vi "get valid output path.vi"(8 "error in (no error)":errorcluster, 11 "TDMS datalogger configuration in":refnum<class "TDMS datalogger configuration.lvclass">) -> (0 "error out":errorcluster, 2 "Path":path, 3 "TDMS datalogger configuration out":refnum<class "TDMS datalogger configuration.lvclass">)   [LabVIEW 2013, in "TDMS datalogger configuration.lvclass"]
uses:
  TDMS datalogger configuration.lvclass
  TDMS datalogger configuration.lvclass/TDMS datalogger configuration.ctl
  <vilib>/NI/Configuration Framework/serializable configuration/NISE_CEF_serializable configuration.lvclass/NISE_CEF_serializable configuration.ctl
  <vilib>/NI/Configuration Framework/serializable configuration/NISE_CEF_serializable configuration.lvclass
  Read Path.vi
  <vilib>/NI/Configuration Framework/serializable configuration/Read UID.vi
panel:
  out "group":string
  out "owner":string
  out "Boolean array":bool[](array[boolean])
  out "permissions":i16
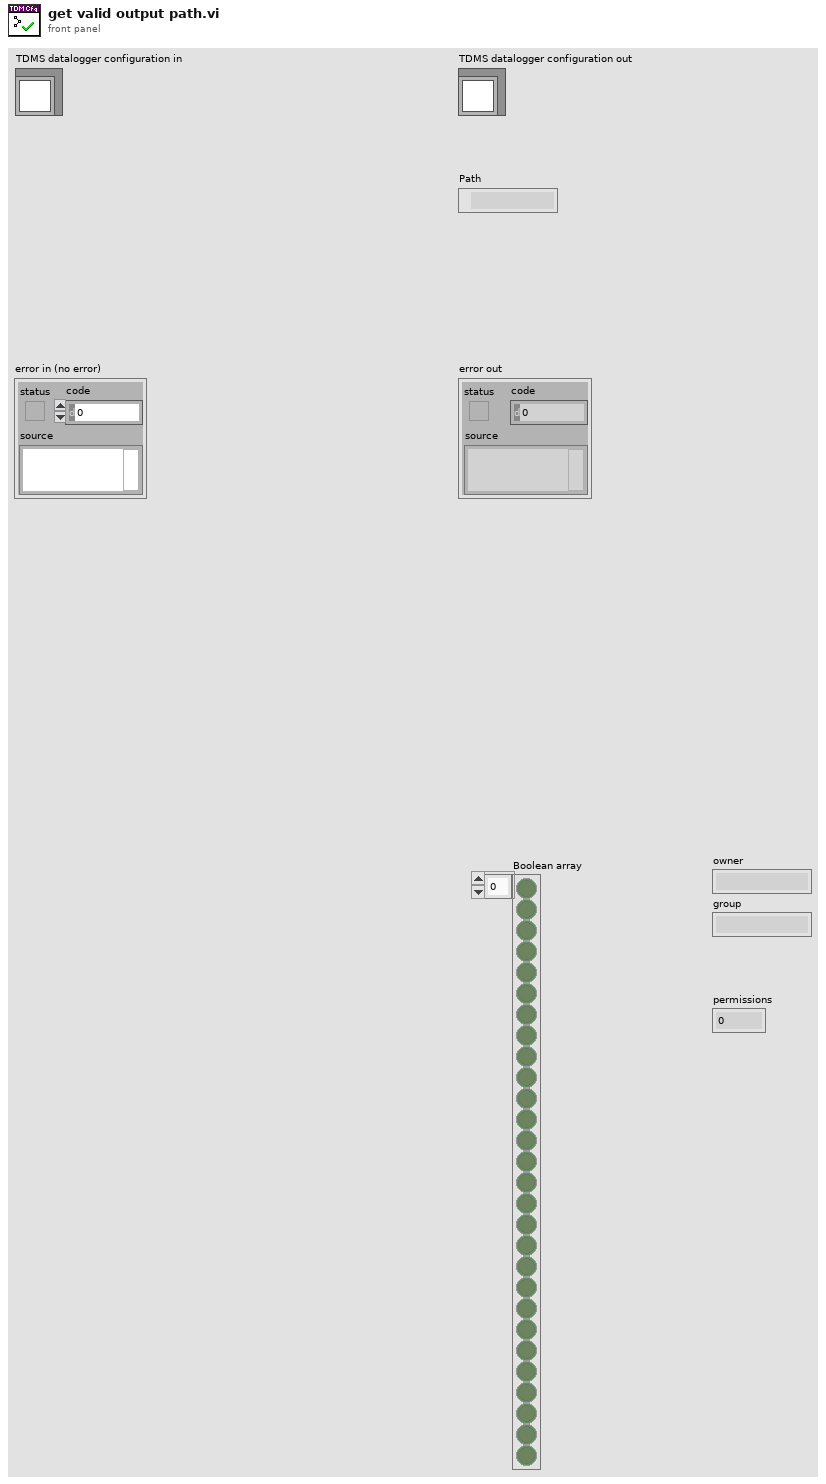
[diagram p1: front panel]
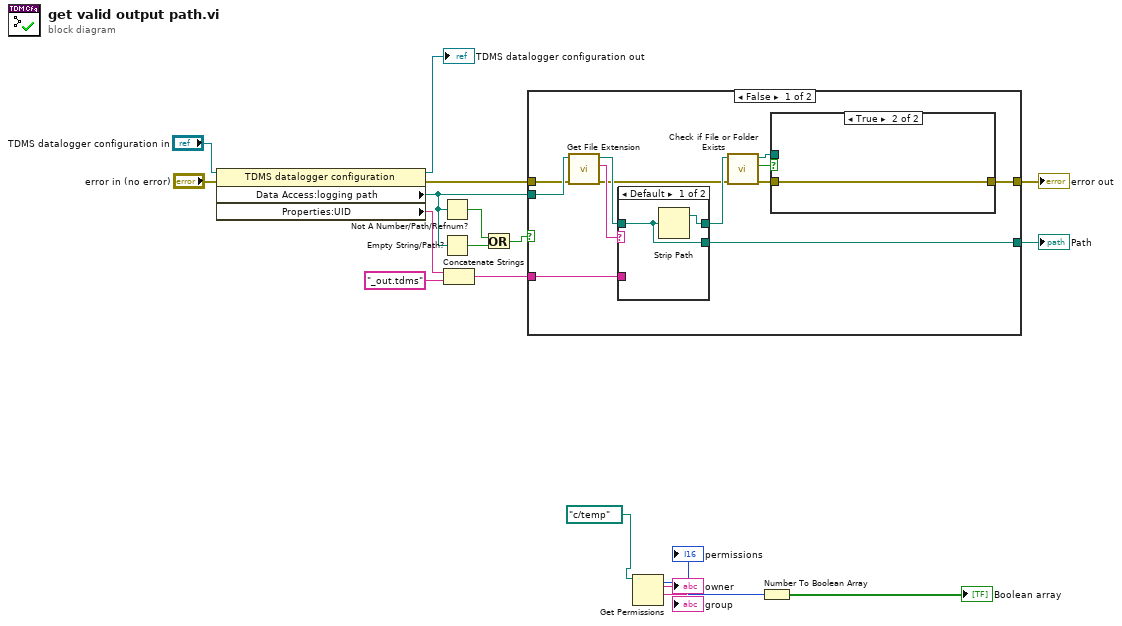
[diagram p0: block diagram]
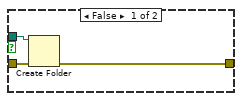
[diagram p2: hidden frame]
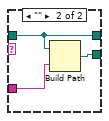
[diagram p3: hidden frame]
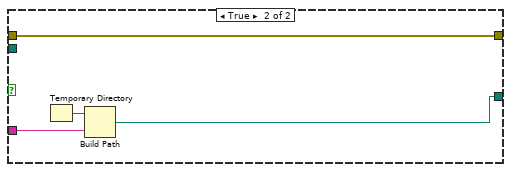
[diagram p4: hidden frame]
diagram:
  n1 = property class="TDMS datalogger configuration"(reference="TDMS datalogger configuration in", error in="error in (no error)") -> (reference out=→"TDMS datalogger configuration out":refnum<class "TDMS datalogger configuration.lvclass">, error out=w15:errorcluster, "Data Access:logging path"=w6:path, "Properties:UID"=w13:string)
  n2 = Not A Number/Path/Refnum?(number/path/refnum=w6) -> (NaN/Path/Refnum?=w17:bool)
  n3 = Empty String/Path?(string/path=w6) -> (empty?=w18:bool)
  n4 = Concatenate Strings(w13, "_out.tdms" ("string")) -> (w12:string)
  n5 = Or(x=w17, y=w18) -> (x .or. y?=w16:bool)
  n6 = case shown="False" w16 {
    tunnel: [w25 w42] -> w11
    tunnel: w6 -> [w30 _]
    tunnel: w15 -> [w29 w40]
    tunnel: w12 -> [w26 w41]
    tunnel: [w21 w40] -> w10
    frame False {
      n7 = call <vilib>:"Get File Extension.vi"("error in (no error)"=w29, "file"=w30) -> ("error out"=w23:errorcluster, "lowercase file extension"=w27:string, "dup file"=w28:path)  [unwired: 6 in, 1 out]
      n8 = case shown="Default" w27 {
        tunnel: w28 -> [w36 w37]
        tunnel: w26 -> [_ w39]
        tunnel: [w36 w38] -> w25
        tunnel: [w35 w37] -> w24
        frame Default {
          n9 = Strip Path(path=w36) -> (stripped path=w35:path)  [unwired: 1 out]
        }
        frame "" {
          n10 = Build Path(base path=w37, name or relative path=w39) -> (appended path=w38:path)
        }
      }
      n11 = call <vilib>:"Check if File or Folder Exists.vi"("error in (no error)"=w23, "path"=w24) -> ("error out"=w20:errorcluster, "file or folder exists?"=w22:bool, "dup path"=w19:path)  [unwired: 7 in]
      n12 = case shown="True" w22 {
        tunnel: [w31 w34] -> w21
        tunnel: w20 -> [w32 w34]
        tunnel: w19 -> [w33 _]
        frame False {
          n13 = Create Folder(path (use dialog)=w33, error in=w32) -> (error out=w31:errorcluster)  [unwired: 1 in, 2 out]
        }
        frame True {
        }
      }
    }
    frame True {
      n14 = Temporary Directory() -> (w43:path)
      n15 = Build Path(base path=w43, name or relative path=w41) -> (appended path=w42:path)
    }
  }
  "error out" <- w10
  "Path" <- w11
  n16 = Get Permissions(11:path "c:/temp" ("path")) -> (1:→"group":string, 2:→"owner":string, 5:w4:i16)  [unwired: 1 in, 2 out]
  "permissions" <- w4
  n17 = Number To Boolean Array(number=w4) -> (Boolean array=→"Boolean array":bool[])
